vi "pmacContorlAndCamera.vi"() -> ()   [LabVIEW 2018]
uses:
  <vilib>/userdefined/High Color/IMAQdx.ctl
  <vilib>/Platform/TimedLoop/XDataNode/timing_clust.ctl
  <vilib>/Platform/TimedLoop/XDataNode/nitl_modes.ctl
  <vilib>/Platform/TimedLoop/XDataNode/wakeup.ctl
  <vilib>/Platform/TimedLoop/XDataNode/XDataNode.xnode
  <vilib>/Platform/TimedLoop/XDataNode/XDNodeRunTimeDep.lvlib
  <vilib>/vision/driver/NI_Vision_Acquisition_Software.lvlib
panel:
  out "拍摄内容":T1(plugin-control)
  in  "中止":bool
  in  "选择相机":T2="cam1"
  in  "PCOMMSERVERLib.IPmacDevice":refnum<k7>
  out "电机1位置":string caption="字符串"
  out "电机2位置":string
  out "电机3位置":string
  out "电机4位置":string
  out "pAnswer 6":string
  out "pstatus 6":i32
  out "下载状态":bool
  in  "error in":errorcluster caption="错误输入"
  out "selected path":path caption="所选路径"
  out "exists":bool caption="存在"
  out "cancelled":bool caption="取消"
  out "error out":errorcluster caption="错误输出"
  in  "错误输入（无错误） 3":errorcluster caption="错误输入（无错误）"
  out "引用输出 7":refnum<k7>
  out "错误输出 3":errorcluster caption="错误输出"
  out "pAnswer 5":string
  out "pstatus 5":i32
  in  "位置":string="0"
  out "pAnswer 4":string
  out "pstatus 4":i32
  in  "错误输入（无错误） 7":errorcluster caption="错误输入（无错误）"
  out "引用输出 6":refnum<k7>
  out "错误输出 7":errorcluster caption="错误输出"
  in  "错误输入（无错误） 6":errorcluster caption="错误输入（无错误）"
  out "引用输出 5":refnum<k7>
  out "错误输出 6":errorcluster caption="错误输出"
  out "pAnswer 3":string
  out "pstatus 3":i32
  out "pAnswer 2":string
  out "pstatus 2":i32
  in  "错误输入（无错误） 5":errorcluster caption="错误输入（无错误）"
  out "引用输出 4":refnum<k7>
  out "错误输出 5":errorcluster caption="错误输出"
  in  "错误输入（无错误） 4":errorcluster caption="错误输入（无错误）"
  out "引用输出 3":refnum<k7>
  out "错误输出 4":errorcluster caption="错误输出"
  out "pAnswer":string
  out "pstatus":i32
  in  "hWindow":i32
  out "引用输出":refnum<k7>
  out "错误输出":errorcluster
  out "选择PMAC卡号":i32
  out "选择状态":bool
  in  "错误输入（无错误） 2":errorcluster caption="错误输入（无错误）"
  out "引用输出 2":refnum<k7>
  out "错误输出 2":errorcluster caption="错误输出"
  out "连接状态":bool
  in  "选择电机":string(combo)="1"
  in  "单步点动":bool
  in  "连接PMAC卡":bool
  in  "正":bool
  in  "停止":bool
  out "执行命令":string
  in  "负":bool
  in  "步长":string="1000"
  in  "killall":bool
  in  "到这":bool
  in  "文件下载":bool
  in  "选择文件":bool
  in  "置零":bool
  in  "发送命令":bool
  in  "命令":string="&1 B1 R"
  # "显示区域"
  # "连接PMAC卡"
  # "ct"
  # "ct"
  # "ct"
  # "ct"
  # "Jog"
  # "ct"
  # "ct"
  # "文件下载"
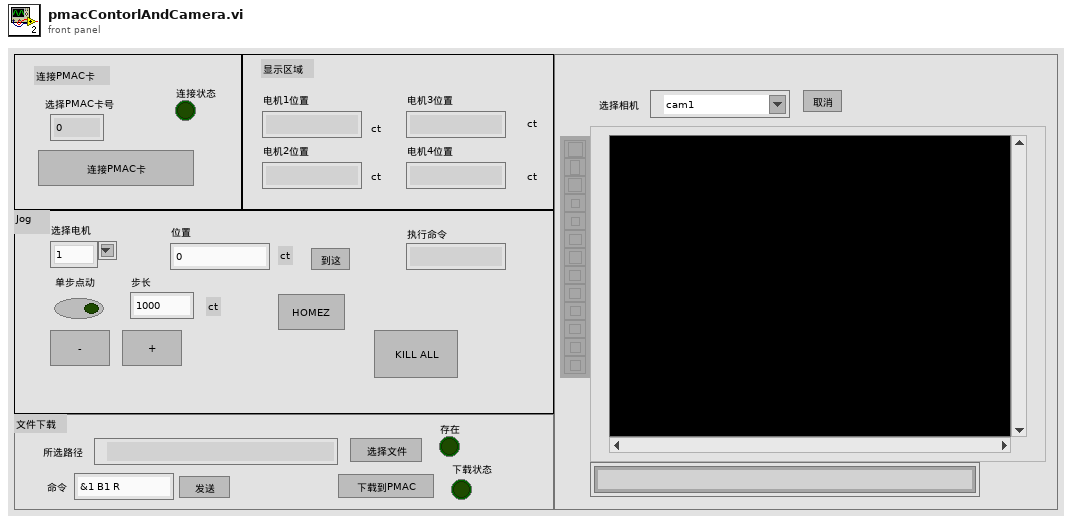
[diagram p1: front panel]
types:
  T1 = typedef "IMAQ Image.ctl" = refnum<image>
  T2 = typedef "IMAQdx.ctl" = refnum<k21>
  T3 = typedef "XDNodeRunTimeDep.lvlib/timing_clust.ctl" = cluster{"Expected End [f-1]":u64, "Actual End [f-1]":u64, "Finished Late? [f-1]":bool, "Expected End [i-1]":u64, "Actual End [i-1]":u64, "Finished Late? [i-1]":bool, "Expected Start [i]":u64, "Actual Start [i]":u64, "Expected Start [f]":u64, "Actual Start [f]":u64, "Source Name":string, "Structure Name":string, "Period":i64, "Deadline":i64, "Offset":i64, "Start":i64, "Priority":i32, "Timeout":i32, "Mode":T4, "Wakeup Reason":T5, "Error":errorcluster, "Source Type":string, "Secondary Source Type":string, "Global End Time":u64, "Global Start Time":u64, "Frame Duration":u64, "Iteration Duration":u64, "Assigned CPU":i32, "I/O Scan Engine Mode":u32}
  T4 = typedef "XDNodeRunTimeDep.lvlib/nitl_modes.ctl" = enum32{"No Change", "Process missed periods, maintain original phase", "Discard missed periods, maintain original phase", "Process missed periods, ignore original phase", "Discard missed periods, ignore original phase"}
  T5 = typedef "XDNodeRunTimeDep.lvlib/wakeup.ctl" = enum32{"Normal", "Aborted", "Asynchronous wakeup", "Timing source error", "Timed loop error", "Timeout"}
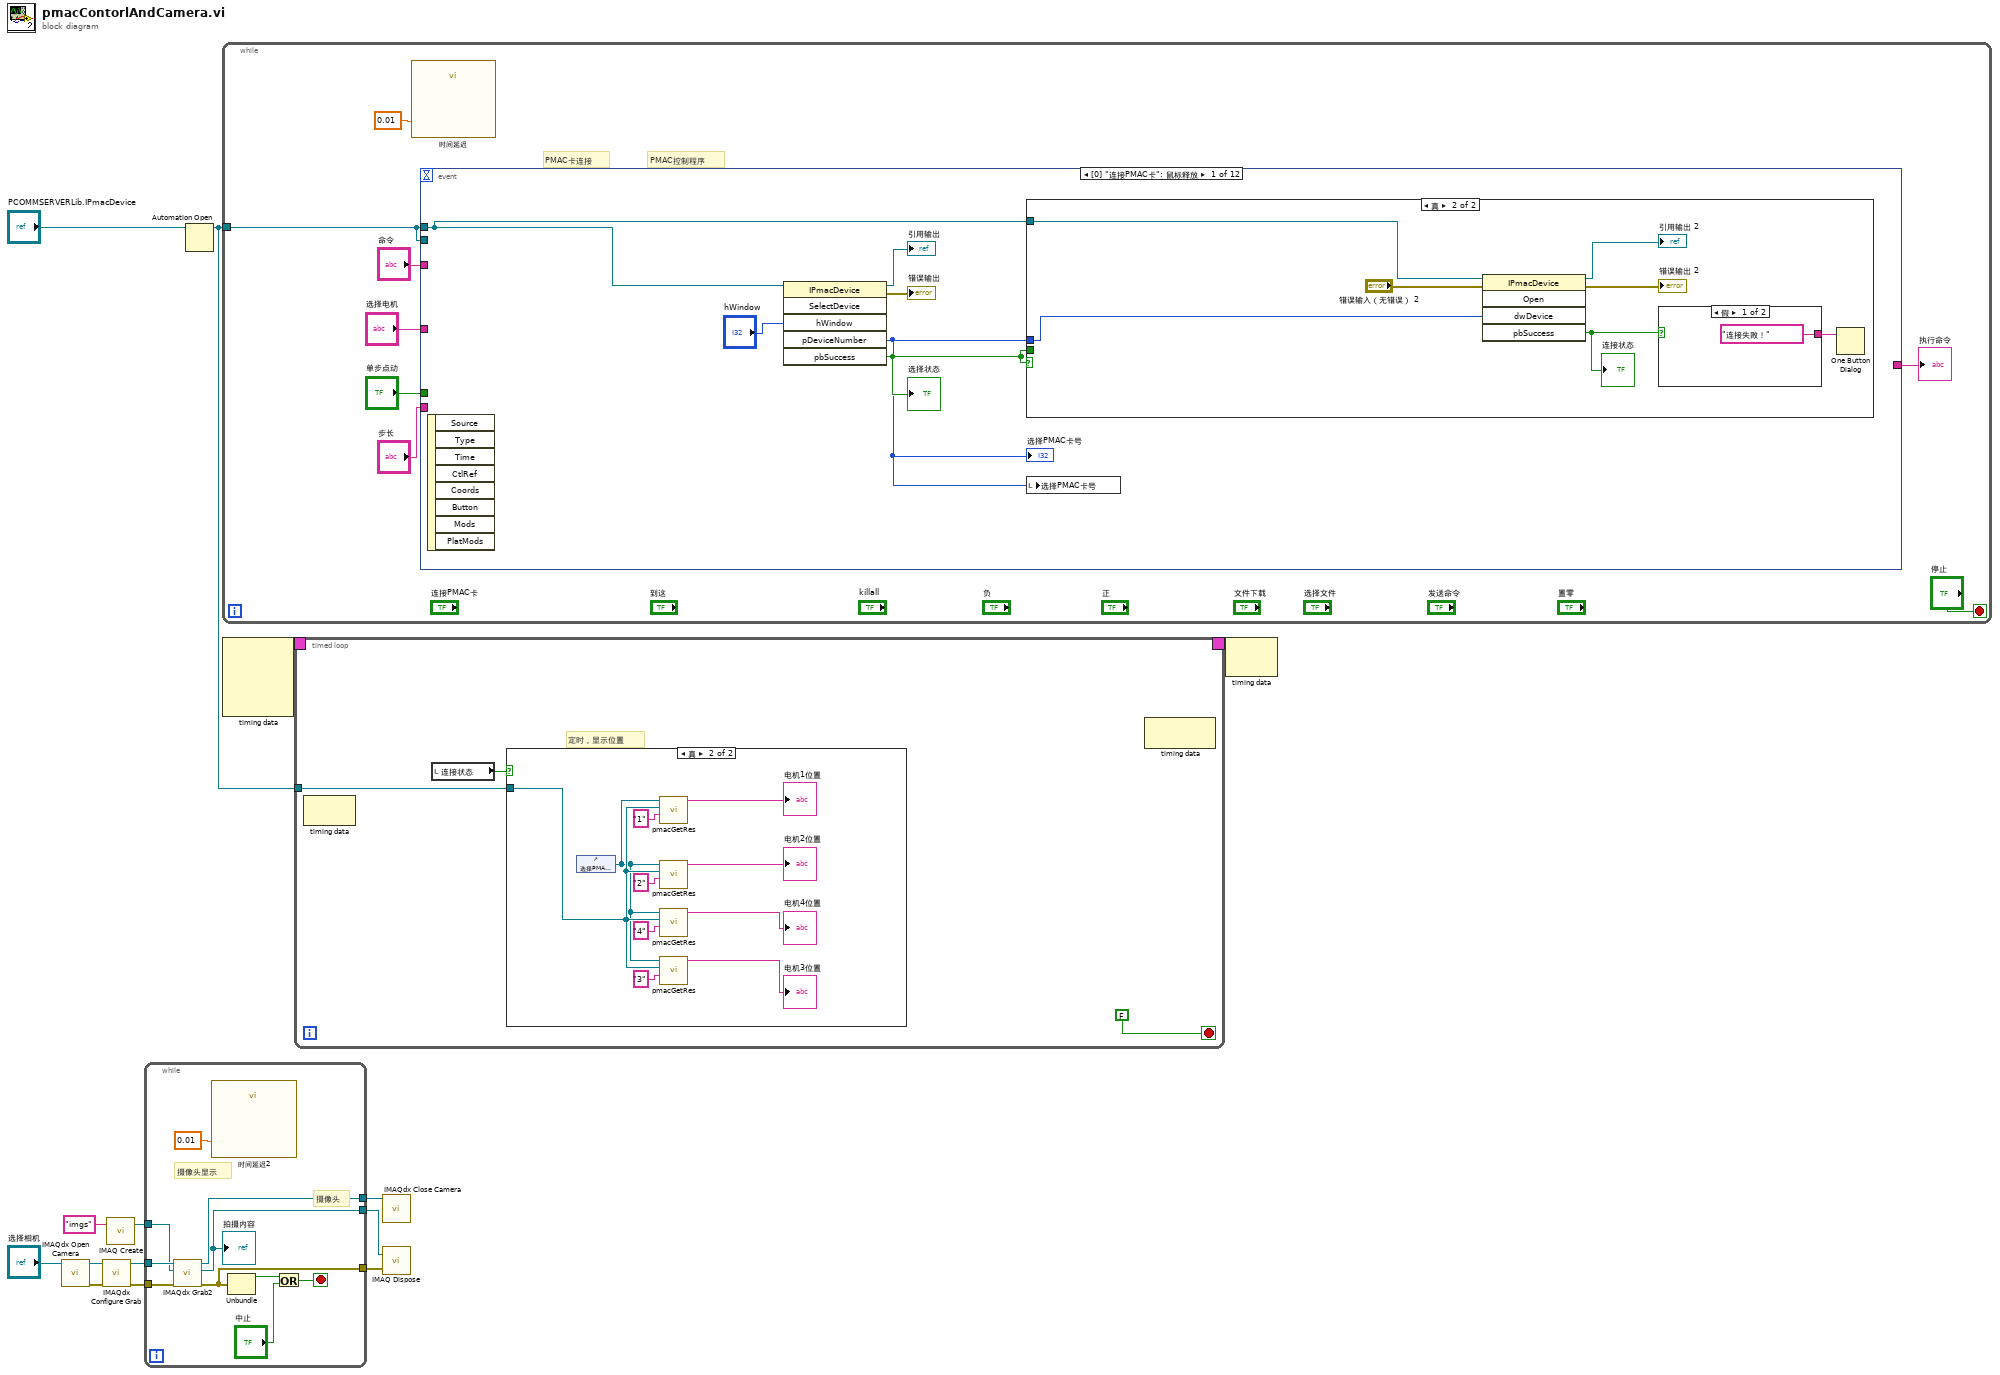
[diagram p0: block diagram]
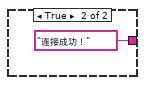
[diagram p4: hidden frame]
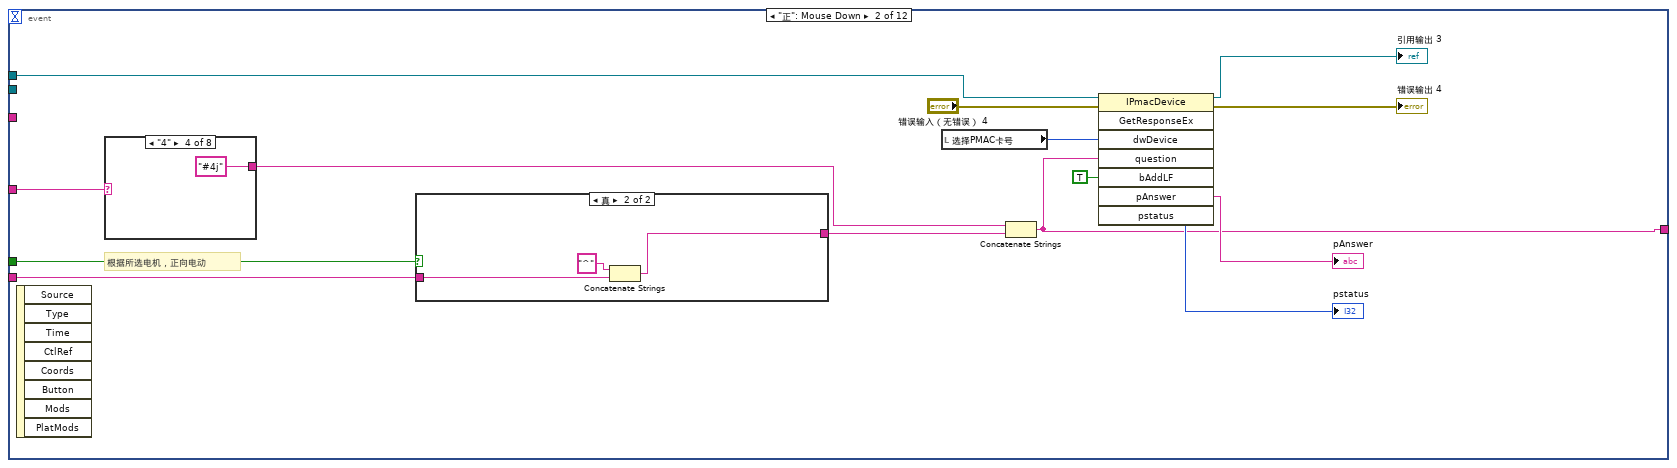
[diagram p5: hidden frame]
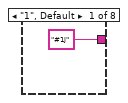
[diagram p6: hidden frame]
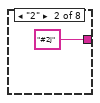
[diagram p7: hidden frame]
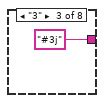
[diagram p8: hidden frame]
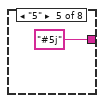
[diagram p9: hidden frame]
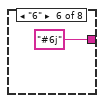
[diagram p10: hidden frame]
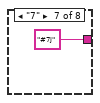
[diagram p11: hidden frame]
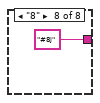
[diagram p12: hidden frame]
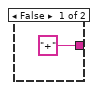
[diagram p13: hidden frame]
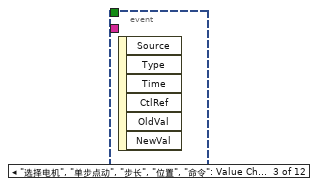
[diagram p14: hidden frame]
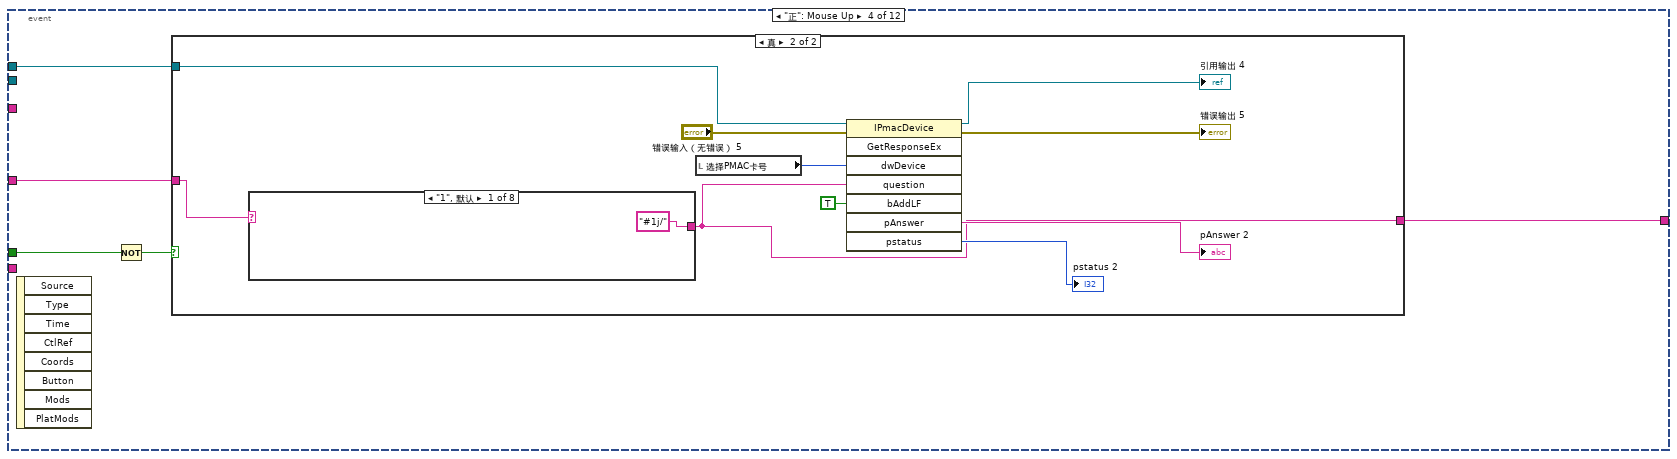
[diagram p15: hidden frame]
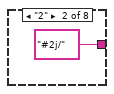
[diagram p17: hidden frame]
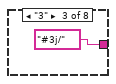
[diagram p18: hidden frame]
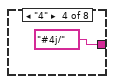
[diagram p19: hidden frame]
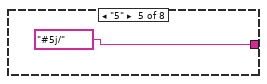
[diagram p20: hidden frame]
diagram:
  n1 = call <vilib>:"IMAQdx Open Camera.vi"("Session In"="选择相机") -> ("error out"=w10:errorcluster, "Session Out"=w9:T2)  [unwired: 9 in]
  n2 = call <vilib>:"IMAQdx Configure Grab.vi"("error in"=w10, "Session In"=w9) -> ("error out"=w8:errorcluster, "Session Out"=w7:T2)  [unwired: 8 in]
  n3 = call "IMAQ Create"("Image Name"="imgs") -> ("New Image"=w4:T1)  [unwired: 4 in, 1 out]
  n4 = while {
    tunnel: w8 -> [w24]
    tunnel: w7 -> [w23]
    tunnel: w4 -> [w22]
    tunnel: [w19] -> w3
    tunnel: [w18] -> w2
    tunnel: [w16] -> w1
    stop <- w21 stop-if-true
    # "摄像头显示"
    # "摄像头"
    n5 = call <vilib>:"IMAQdx Grab2.vi"("error in"=w24, "Image In"=w22, "Session In"=w23) -> ("error out"=w16:errorcluster, "Image Out"=w18:T1, "Session Out"=w19:T2)  [unwired: 5 in, 1 out]
    "拍摄内容" <- w18
    n6 = call "时间延迟2"("Delay Time (s)"=0.01) -> ()  [unwired: 10 in, 1 out]
    n7 = Unbundle(w16) -> ("status"=w17:bool)  [unwired: 2 out]
    n8 = Or(x=w17, y="中止") -> (x .or. y?=w21:bool)
  }
  n9 = Automation Open(Automation Refnum="PCOMMSERVERLib.IPmacDevice") -> (Automation Refnum=w11:refnum<k7>)  [unwired: 3 in, 1 out]
  n10 = while {
    tunnel: w11 -> [w27]
    stop <- "停止" stop-if-true
    # "PMAC控制程序"
    # "PMAC卡连接"
    n11 = call "时间延迟"("Delay Time (s)"=0.01) -> ()  [unwired: 10 in, 1 out]
    n12 = event shown="[0] \"连接PMAC卡\": 鼠标释放" {
      selector: _ -> [_ _ _ _ _ _ _ _ _ _ _ _]
      dyn-events: _ -> [_ _ _ _ _ _ _ _ _ _ _ _]
      timeout: _ -> [_ _ _ _ _ _ _ _ _ _ _ _]
      tunnel: "选择电机" -> [_ w53 _ w76 w100 w126 _ w169 _ _ w209 _]
      tunnel: "单步点动" -> [_ w52 _ w77 w99 w125 _ _ _ _ _ _]
      tunnel: w27 -> [w33 w50 _ w75 w101 w124 _ w176 _ w194 _ w223]
      tunnel: [_ w49 _ w74 w97 w123 w147 w165 _ _ w204 w221] -> w29
      tunnel: "步长" -> [_ w48 _ _ w98 _ _ _ _ _ _ _]
      tunnel: w27 -> [_ _ _ _ _ _ w148 _ _ _ w207 _]
      tunnel: "命令" -> [_ _ _ _ _ _ _ _ _ _ _ w222]
      event "连接PMAC卡": Mouse Up {
        n13 = event-data() -> ()  [unwired: 1 in, 8 out]
        n14 = invoke class="IPmacDevice" method="SelectDevice"(reference=w33, "hWindow"="hWindow") -> (reference out=→"引用输出":refnum<k7>, error out=→"错误输出":errorcluster, "pDeviceNumber"=w34:i32, "pbSuccess"=w35:bool)  [unwired: 4 in, 2 out]
        "选择PMAC卡号" <- w34
        "选择状态" <- w35
        n15 = case shown="真" w35 {
          tunnel: w35 -> [_ _]
          tunnel: w34 -> [_ w42]
          tunnel: w33 -> [_ w41]
          frame False {
          }
          frame True {
            n16 = invoke class="IPmacDevice" method="Open"(reference=w41, error in="错误输入（无错误） 2", "dwDevice"=w42) -> (reference out=→"引用输出 2":refnum<k7>, error out=→"错误输出 2":errorcluster, "pbSuccess"=w39:bool)  [unwired: 2 in, 2 out]
            "连接状态" <- w39
            n17 = case shown="假" w39 {
              tunnel: ["连接失败！" "连接成功！"] -> w40
              frame False {
              }
              frame True {
              }
            }
            n18 = One Button Dialog(message=w40) -> ()  [unwired: 1 in, 1 out]
          }
        }
        n19 = local write "选择PMAC卡号"(w34) -> ()
      }
      event "正": Mouse Down {
        # "根据所选电机，正向电动"
        n20 = event-data() -> ()  [unwired: 1 in, 8 out]
        n21 = case "条件结构" shown="\"4\"" w53 {
          tunnel: ["#1j" "#2j" "#3j" "#4j" "#5j" "#6j" "#7j" "#8j"] -> w55
          frame "1", Default {
          }
          frame "2" {
          }
          frame "3" {
          }
          frame "4" {
          }
          frame "5" {
          }
          frame "6" {
          }
          frame "7" {
          }
          frame "8" {
          }
        }
        n22 = case shown="真" w52 {
          tunnel: ["+" w72] -> w56
          tunnel: w48 -> [_ w71]
          frame False {
          }
          frame True {
            n23 = Concatenate Strings("^", w71) -> (w72:string)
          }
        }
        n24 = local read "选择PMAC卡号"() -> (w51:i32)
        n25 = Concatenate Strings(w55, w56) -> (w49:string)
        n26 = invoke class="IPmacDevice" method="GetResponseEx"(reference=w50, error in="错误输入（无错误） 4", "dwDevice"=w51, "question"=w49, "bAddLF"=TRUE) -> (reference out=→"引用输出 3":refnum<k7>, error out=→"错误输出 4":errorcluster, "pAnswer"=→"pAnswer":string, "pstatus"=→"pstatus":i32)  [unwired: 3 in, 4 out]
      }
      event "选择电机", "单步点动", "步长", "位置", "命令": Value Change {
        n27 = event-data() -> ()  [unwired: 1 in, 6 out]
      }
      event "正": Mouse Up {
        n28 = event-data() -> ()  [unwired: 1 in, 8 out]
        n29 = Not(x=w77) -> (.not. x?=w78:bool)
        n30 = case shown="真" w78 {
          tunnel: w75 -> [_ w82]
          tunnel: w76 -> [_ w81]
          tunnel: [_ w79] -> w74
          frame False {
          }
          frame True {
            n31 = case shown="\"1\", 默认" w81 {
              tunnel: ["#1j/" "#2j/" "#3j/" "#4j/" "#5j/" "#6j/" "#7j/" "#8j/"] -> w79
              frame "1", Default {
              }
              frame "2" {
              }
              frame "3" {
              }
              frame "4" {
              }
              frame "5" {
              }
              frame "6" {
              }
              frame "7" {
              }
              frame "8" {
              }
            }
            n32 = local read "选择PMAC卡号"() -> (w80:i32)
            n33 = invoke class="IPmacDevice" method="GetResponseEx"(reference=w82, error in="错误输入（无错误） 5", "dwDevice"=w80, "question"=w79, "bAddLF"=TRUE) -> (reference out=→"引用输出 4":refnum<k7>, error out=→"错误输出 5":errorcluster, "pAnswer"=→"pAnswer 2":string, "pstatus"=→"pstatus 2":i32)  [unwired: 3 in, 4 out]
          }
        }
      }
      event "负": Mouse Down {
        n34 = event-data() -> ()  [unwired: 1 in, 8 out]
        n35 = case "条件结构" shown="\"4\"" w100 {
          tunnel: ["#1j" "#2j" "#3j" "#4j" "#5j" "#6j" "#7j" "#8j"] -> w104
          frame "1", Default {
          }
          frame "2" {
          }
          frame "3" {
          }
          frame "4" {
          }
          frame "5" {
          }
          frame "6" {
          }
          frame "7" {
          }
          frame "8" {
          }
        }
        n36 = case shown="真" w99 {
          tunnel: ["-" w121] -> w105
          tunnel: w98 -> [_ w120]
          frame False {
          }
          frame True {
            n37 = Concatenate Strings("^-", w120) -> (w121:string)
          }
        }
        n38 = local read "选择PMAC卡号"() -> (w102:i32)
        n39 = Concatenate Strings(w104, w105) -> (w97:string)
        n40 = invoke class="IPmacDevice" method="GetResponseEx"(reference=w101, error in="错误输入（无错误） 6", "dwDevice"=w102, "question"=w97, "bAddLF"=TRUE) -> (reference out=→"引用输出 5":refnum<k7>, error out=→"错误输出 6":errorcluster, "pAnswer"=→"pAnswer 3":string, "pstatus"=→"pstatus 3":i32)  [unwired: 3 in, 4 out]
      }
      event "负": Mouse Up {
        n41 = event-data() -> ()  [unwired: 1 in, 8 out]
        n42 = Not(x=w125) -> (.not. x?=w127:bool)
        n43 = case shown="真" w127 {
          tunnel: w124 -> [_ w131]
          tunnel: w126 -> [_ w130]
          tunnel: [_ w128] -> w123
          frame False {
          }
          frame True {
            n44 = case shown="\"5\"" w130 {
              tunnel: ["#1j/" "#2j/" "#3j/" "#4j/" "#5j/" "#6j/" "#7j/" "#8j/"] -> w128
              frame "1", Default {
              }
              frame "2" {
              }
              frame "3" {
              }
              frame "4" {
              }
              frame "5" {
              }
              frame "6" {
              }
              frame "7" {
              }
              frame "8" {
              }
            }
            n45 = local read "选择PMAC卡号"() -> (w129:i32)
            n46 = invoke class="IPmacDevice" method="GetResponseEx"(reference=w131, error in="错误输入（无错误） 7", "dwDevice"=w129, "question"=w128, "bAddLF"=TRUE) -> (reference out=→"引用输出 6":refnum<k7>, error out=→"错误输出 7":errorcluster, "pAnswer"=→"pAnswer 4":string, "pstatus"=→"pstatus 4":i32)  [unwired: 3 in, 4 out]
          }
        }
      }
      event "killall": Mouse Up {
        n47 = event-data() -> ()  [unwired: 1 in, 8 out]
        n48 = case shown="真" TRUE {
          tunnel: w148 -> [_ w150]
          tunnel: [_ w149] -> w147
          frame False {
          }
          frame True {
            w149 = "K"
            n49 = for {
              N: 4 -> [_]
              tunnel: w150 -> [w163]
              i -> [w160]
              n50 = Add(x=w160, y=1) -> (x+y=w158:i32)
              n51 = Number To Decimal String(number=w158) -> (decimal integer string=w157:string)  [unwired: 1 in]
              n52 = Concatenate Strings("#", w157, "j/") -> (w154:string)
              n53 = local read "选择PMAC卡号"() -> (w162:i32)
              n54 = invoke class="IPmacDevice" method="GetResponseEx"(reference=w163, "dwDevice"=w162, "question"=w154, "bAddLF"=TRUE) -> ()  [unwired: 4 in, 8 out]
            }
            n55 = local read "选择PMAC卡号"() -> (w153:i32)
            n56 = invoke class="IPmacDevice" method="GetResponseEx"(reference=w150, "dwDevice"=w153, "question"=w149, "bAddLF"=TRUE) -> ()  [unwired: 4 in, 8 out]
          }
        }
      }
      event "到这": Value Change {
        n57 = event-data() -> ()  [unwired: 1 in, 6 out]
        n58 = case shown="\"5\"" w169 {
          tunnel: ["#1j" "#2j" "#3j" "#4j" "#5j" "#6j" "#7j" "#8j"] -> w168
          frame "1", Default {
          }
          frame "2" {
          }
          frame "3" {
          }
          frame "4" {
          }
          frame "5" {
          }
          frame "6" {
          }
          frame "7" {
          }
          frame "8" {
          }
        }
        n59 = local read "选择PMAC卡号"() -> (w164:i32)
        n60 = Concatenate Strings(w168, "=", "位置") -> (w165:string)
        n61 = invoke class="IPmacDevice" method="GetResponseEx"(reference=w176, error in="错误输入（无错误） 3", "dwDevice"=w164, "question"=w165, "bAddLF"=TRUE) -> (reference out=→"引用输出 7":refnum<k7>, error out=→"错误输出 3":errorcluster, "pAnswer"=→"pAnswer 5":string, "pstatus"=→"pstatus 5":i32)  [unwired: 3 in, 4 out]
      }
      event "选择文件": Mouse Up {
        n62 = event-data() -> ()  [unwired: 1 in, 8 out]
        n63 = call "文件对话框"("default name"="请选择文件", "error in"="error in", "pattern (all files)"="*.txt;*.pmc", "pattern label"="ACLII") -> ("selected path"=→"selected path":path, "exists"=→"exists":bool, "cancelled"=→"cancelled":bool, "error out"=→"error out":errorcluster)  [unwired: 8 in]
      }
      event "文件下载": Mouse Up {
        n64 = event-data() -> ()  [unwired: 1 in, 8 out]
        n65 = local read "exists"() -> (w193:bool)
        n66 = case shown="真" w193 {
          tunnel: w194 -> [_ w197]
          frame False {
          }
          frame True {
            n67 = local read "selected path"() -> (w195:path)
            n68 = local read "选择PMAC卡号"() -> (w196:i32)
            n69 = Path To String(path=w195) -> (string=w203:string)
            n70 = invoke class="IPmacDevice" method="Download"(reference=w197, "dwDevice"=w196, "filePath"=w203, "bMacro"=TRUE, "bMap"=TRUE, "bLog"=TRUE, "bDnld"=TRUE) -> ("pbSuccess"=→"下载状态":bool)  [unwired: 3 in, 9 out]
          }
        }
      }
      event "置零": Mouse Up {
        n71 = event-data() -> ()  [unwired: 1 in, 8 out]
        n72 = case shown="\"1\", 默认" w209 {
          tunnel: ["#1" "#2" "#3" "#4" "#5" "#6" "#7" "#8"] -> w211
          frame "1", Default {
          }
          frame "2" {
          }
          frame "3" {
          }
          frame "4" {
          }
          frame "5" {
          }
          frame "6" {
          }
          frame "7" {
          }
          frame "8" {
          }
        }
        n73 = local read "选择PMAC卡号"() -> (w208:i32)
        n74 = Concatenate Strings(w211, "HOMEZ") -> (w204:string)
        n75 = invoke class="IPmacDevice" method="GetResponseEx"(reference=w207, "dwDevice"=w208, "question"=w204, "bAddLF"=TRUE) -> ("pAnswer"=→"pAnswer 6":string, "pstatus"=→"pstatus 6":i32)  [unwired: 4 in, 6 out]
      }
      event "发送命令": Mouse Up {
        n76 = event-data() -> ()  [unwired: 1 in, 8 out]
        n77 = String Length(string=w222) -> (length=w224:i32)
        n78 = case shown="1, 默认" w224 {
          tunnel: w223 -> [_ w227]
          tunnel: w222 -> [_ w225]
          tunnel: [_ w225] -> w221
          frame 0 {
          }
          frame 1, Default {
            n79 = local read "选择PMAC卡号"() -> (w228:i32)
            n80 = invoke class="IPmacDevice" method="GetResponseEx"(reference=w227, "dwDevice"=w228, "question"=w225, "bAddLF"=TRUE) -> ()  [unwired: 4 in, 8 out]
          }
        }
      }
    }
    "执行命令" <- w29
  }
  n81 = node-c288() -> (w14:T3)  [unwired: 4 in]
  n82 = timed-loop {
    timing: w14 -> [_]
    timing-out: [_] -> w13
    tunnel: w11 -> [w231]
    stop <- FALSE stop-if-true
    # "定时，显示位置"
    n83 = node-c288() -> ()  [unwired: 1 in, 1 out]
    n84 = local read "连接状态"() -> (w230:bool)
    n85 = case shown="真" w230 {
      tunnel: w231 -> [_ w235]
      frame False {
      }
      frame True {
        n86 = control-ref of="选择PMAC卡号"() -> (w232:refnum<vi>)
        n87 = call "pmacGetRes.vi"("字符串"="1", "PCOMMSERVERLib.IPmacDevice"=w235, "Digital输入"=w232) -> ("pAnswer"=→"电机1位置":string)  [unwired: 8 in]
        n88 = call "pmacGetRes.vi"("字符串"="2", "PCOMMSERVERLib.IPmacDevice"=w235, "Digital输入"=w232) -> ("pAnswer"=→"电机2位置":string)  [unwired: 8 in]
        n89 = call "pmacGetRes.vi"("字符串"="4", "PCOMMSERVERLib.IPmacDevice"=w235, "Digital输入"=w232) -> ("pAnswer"=→"电机4位置":string)  [unwired: 8 in]
        n90 = call "pmacGetRes.vi"("字符串"="3", "PCOMMSERVERLib.IPmacDevice"=w235, "Digital输入"=w232) -> ("pAnswer"=→"电机3位置":string)  [unwired: 8 in]
      }
    }
    n91 = node-c288() -> ()  [unwired: 1 in, 1 out]
  }
  n92 = call <vilib>:"IMAQdx Close Camera.vi"("Session In"=w3) -> ()  [unwired: 10 in, 1 out]
  n93 = call "IMAQ Dispose"("Image"=w2, "error in (no error)"=w1) -> ()  [unwired: 4 in, 1 out]
  n94 = node-c288(w13) -> ()  [unwired: 1 out]
